vi "ex_createorOpenTDM.vi"(0 "file path in":path, 1 "overwrite_mode_multi":T3(ring), 2 "overwrite_mode":T4(ring), 3 "append info in":T5, 4 "file dialog?":bool, 5 "error in (no error)":errorcluster, 6 "file params":T1 {"Flags"."time preference" items=["Absolute", "Relative"]; "Flags"."x_columns" items=["None", "One", "Multiple"]; "origin time" format="%<%X\n%x>T"}, 7 "multi_file":bool, 9 "new file?":bool, 11 "Simulate Non-First Call":bool) -> (13 "new file was created":bool, 14 "file path out":path, 15 "dialog was cancelled":bool, 16 "keep loop going":bool, 17 "append info out":T5, 18 "file params out":T1 {"Flags"."time preference" items=["Absolute", "Relative"]; "Flags"."x_columns" items=["None", "One", "Multiple"]; "origin time" format="%<%X\n%x>T"}, 19 "error out":errorcluster)   [LabVIEW 2017]
uses:
  <vilib>/Platform/express/TDMExpress.llb/ex_appendInfoTDM.ctl
  <vilib>/express/express output/ExFileWriteBlock.llb/ex_WriteFileParams.ctl
  <vilib>/express/express input/ExFileReadBlock.llb/ex_ReadFileParams.ctl
  <vilib>/Platform/storage/lvStorage.llb/_openFunction.ctl
  <vilib>/express/express shared/ExFile.llb/ex_FileFormatSelector.ctl
  <vilib>/express/express shared/ExFile.llb/ex_FileGlobals.vi
  <vilib>/Platform/storage/Storage.llb/__closeStorageFromObject.vi
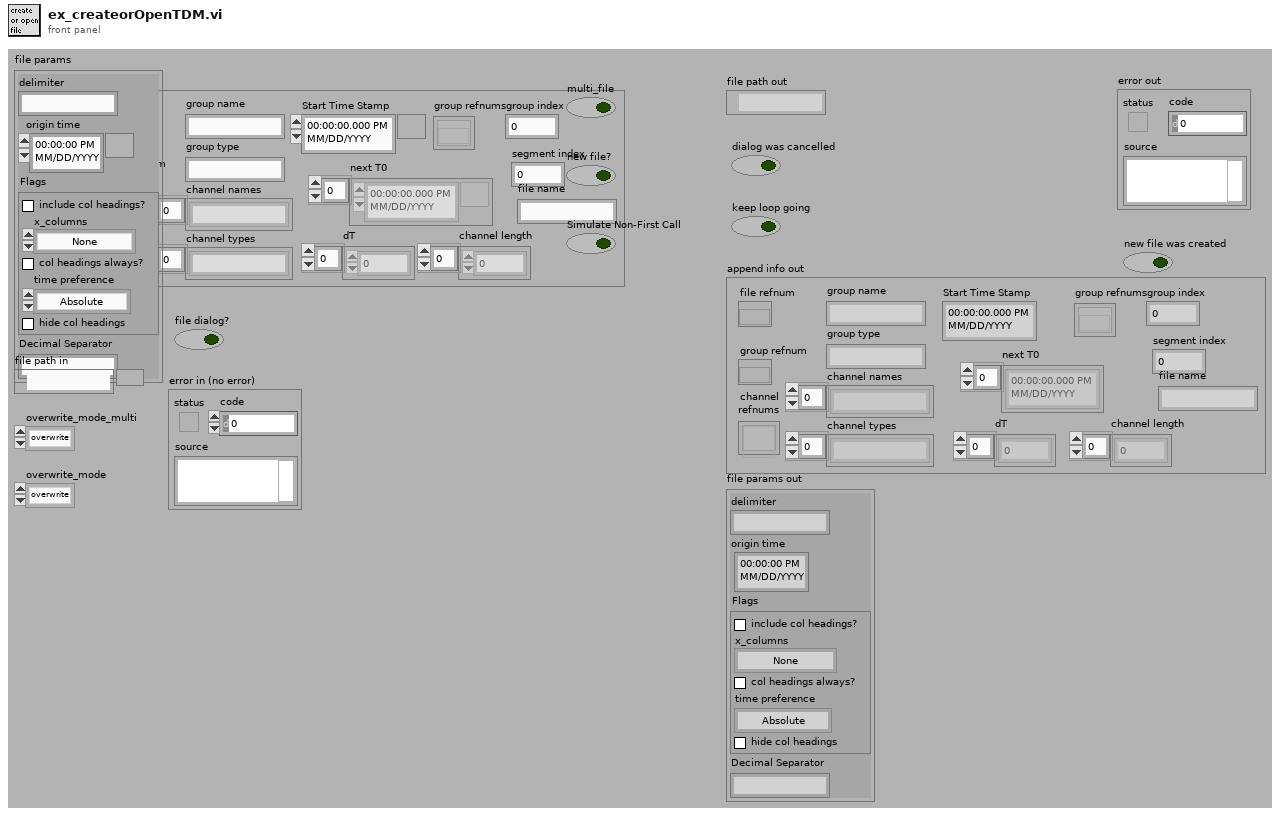
[diagram p1: front panel]
types:
  T1 = typedef "ex_WriteFileParams.ctl" = cluster{"delimiter":string, "origin time":timestamp, "Flags":T2, "Decimal Separator":string}
  T2 = typedef "ex_ReadFileParams.ctl" = cluster{"include col headings?":bool, "x_columns":u16, "col headings always?":bool, "time preference":u16, "hide col headings":bool}
  T3 = enum16{"overwrite", "overwrite & backup", "next avail"}
  T4 = enum16{"overwrite", "overwrite & backup", "append", "next avail"}
  T5 = typedef "ex_appendInfoTDM.ctl" = cluster{"channel\nrefnums":refnum<k20>[], "channel names":string[], "channel types":string[], "file refnum":refnum<k20>, "group refnum":refnum<k20>, "group name":string, "group type":string, "next T0":timestamp[], "dT":dbl[], "Start Time Stamp":timestamp, "channel length":u32[], "group index":u32, "group refnums":refnum<k20>[], "file name":string, "segment index":u32}
  T6 = typedef "ex_FileFormatSelector.ctl" = enum32{"lvm", "tdm", "other"}
  T7 = typedef "_openFunction.ctl" = enum16{"open", "open or create", "create or replace", "create", "open (read only)"}
  T8 = enum16{"existing file", "new file", "new or existing file", "existing dir", "new dir", "new or existing dir", "existing file (use LLBs)", "new file (use LLBs)", "new or existing file (use LLBs)", "new or existing file or directory (use LLBs)"}
  T9 = cluster{"message":string, "T button name":string, "F button name":string}
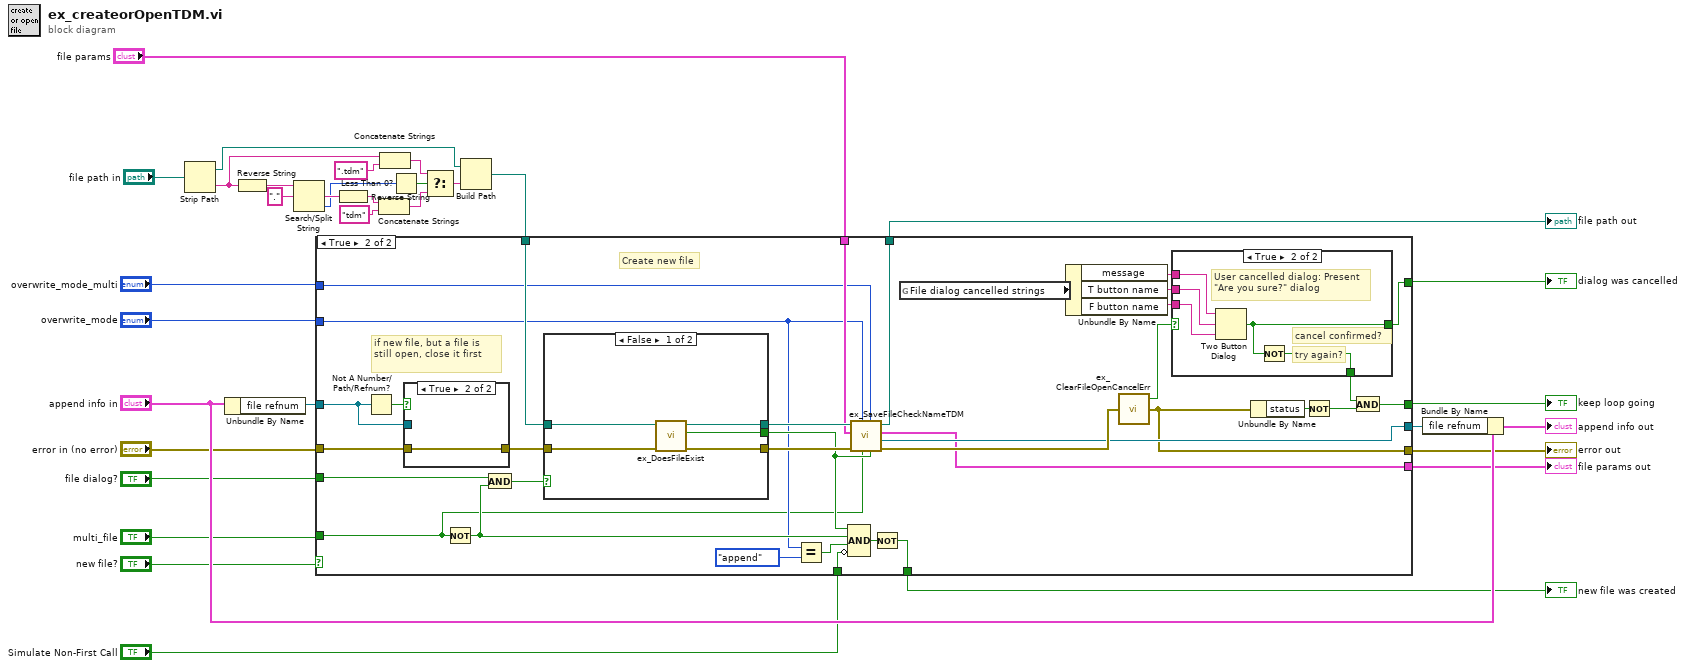
[diagram p0: block diagram]
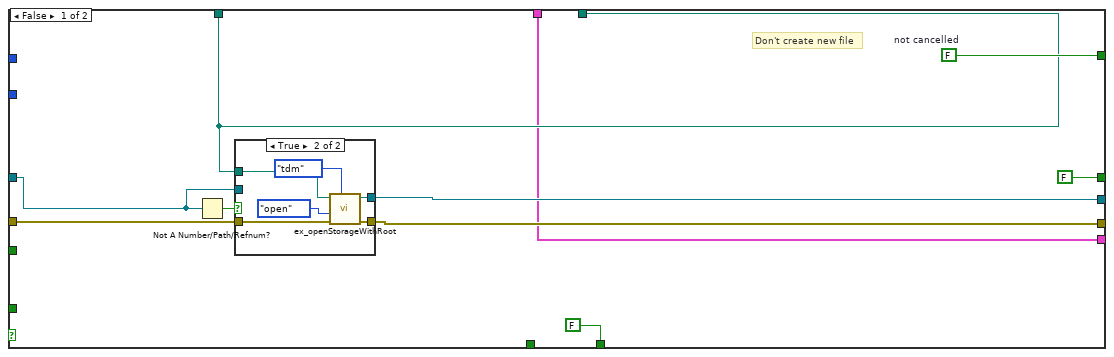
[diagram p2: hidden frame]
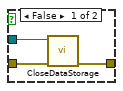
[diagram p4: hidden frame]
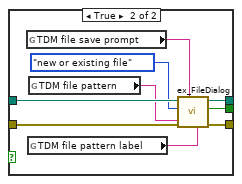
[diagram p6: hidden frame]
diagram:
  n1 = Strip Path(path="file path in") -> (stripped path=w3:path, name=w5:string)
  n2 = Unbundle By Name("append info in") -> ("file refnum"=w28:refnum<k20>)
  n3 = Reverse String(1:w5) -> (0:w15:string)
  n4 = Search/Split String(string=w15, search string/char (-)=".") -> (match + rest of string=w13:string, offset of match=w10:i32)  [unwired: 2 out]
  n5 = Reverse String(1:w13) -> (0:w11:string)
  n6 = Concatenate Strings(w11, "tdm" ("replace string (\"\")")) -> (w6:string)
  n7 = Concatenate Strings(w5, ".tdm" ("replace string (\"\")")) -> (w7:string)
  n8 = Less Than 0?(x=w10) -> (x < 0?=w9:bool)
  n9 = Select(t=w7, s=w9, f=w6) -> (s? t:f=w4:string)
  n10 = Build Path(base path=w3, name or relative path=w4) -> (appended path=w1:path)
  n11 = case shown="True" "new file?" {
    tunnel: "error in (no error)" -> [w40 w58]
    tunnel: w1 -> [w37 w78]
    tunnel: [w39 w61] -> w26
    tunnel: [w34 w53] -> w27
    tunnel: "Simulate Non-First Call" -> [_ w76]
    tunnel: [w43 w72] -> w24
    tunnel: [FALSE w71] -> w30
    tunnel: [w38 w68] -> w32
    tunnel: "file params" -> [w34 w67]
    tunnel: "multi_file" -> [_ w52]
    tunnel: "file dialog?" -> [_ w66]
    tunnel: "overwrite_mode_multi" -> [_ w65]
    tunnel: "overwrite_mode" -> [_ w64]
    tunnel: [FALSE w59] -> w23
    tunnel: w28 -> [w35 w55]
    tunnel: [w37 w54] -> w25
    frame False {
      w43 = FALSE  # not cancelled
      # "Don't create new file"
      n12 = Not A Number/Path/Refnum?(number/path/refnum=w35) -> (NaN/Path/Refnum?=w36:bool)
      n13 = case shown="True" w36 {
        tunnel: w40 -> [w45 w50]
        tunnel: [w45 w49] -> w39
        tunnel: [w44 w48] -> w38
        tunnel: w37 -> [_ w47]
        tunnel: w35 -> [w44 _]
        frame False {
        }
        frame True {
          n14 = call <vilib>:"ex_openStorageWithRoot.vi"("storage_format"=ex_FileFormatSelector."tdm", "error in (no error)"=w50, "Overwrite Options"=_openFunction."open", "Storage Location"=w47) -> ("error out"=w49:errorcluster, "Data Object"=w48:refnum<k20>)  [unwired: 1 in, 5 out]
        }
      }
    }
    frame True {
      # "if new file, but a file is still open, close it first"
      # "Create new file"
      n15 = Not A Number/Path/Refnum?(number/path/refnum=w55) -> (NaN/Path/Refnum?=w56:bool)
      n16 = case shown="True" w56 {
        tunnel: w58 -> [w89 w90]
        tunnel: [w88 w90] -> w57
        tunnel: w55 -> [w87 _]
        frame False {
          n17 = call-poly <vilib>:"CloseDataStorage.vi"("error in (no error)"=w89, "storage refnum"=w87) -> ("error out"=w88:errorcluster)  [unwired: 5 out]
        }
        frame True {
        }
      }
      n18 = Not(x=w52) -> (.not. x?=w86:bool)
      n19 = And(x=w66, y=w86) -> (x .and. y?=w85:bool)
      n20 = case shown="False" w85 {
        tunnel: w78 -> [w100 w110]
        tunnel: [w99 w109] -> w74
        tunnel: [w98 w108] -> w75
        tunnel: w57 -> [w101 w107]
        tunnel: [w97 w106] -> w73
        frame False {
          n21 = call <vilib>:"ex_DoesFileExist.vi"("error in"=w101, "file path"=w100) -> ("error out"=w98:errorcluster, "file exists"=w97:bool, "dup file path"=w99:path)  [unwired: 3 out]
        }
        frame True {
          n22 = global read "ex_FileGlobals.vi" "TDM file save prompt"() -> (w104:string)
          n23 = global read "ex_FileGlobals.vi" "TDM file pattern label"() -> (w103:string)
          n24 = global read "ex_FileGlobals.vi" "TDM file pattern"() -> (w102:string)
          n25 = call <vilib>:"ex_FileDialog.vi"("pattern label"=w103, "pattern"=w102, "prompt"=w104, "error in (no error)"=w107, "select mode"=T8."new or existing file", "start path"=w110) -> ("error out"=w108:errorcluster, "file exists?"=w106:bool, "selected file path"=w109:path)  [unwired: 3 out]
        }
      }
      n26 = Equal?(x=w64, y=T4."append" ("overwrite_mode")) -> (x = y?=w80:bool)
      n27 = Compound Arithmetic op=AND(w73, w86, w80, invert w76) -> (w79:bool)
      n28 = call <vilib>:"ex_SaveFileCheckNameTDM.vi"("file exists?"=w73, "overwrite_mode_multi"=w65, "multi_file"=w52, "overwrite_mode"=w64, "error in (no error)"=w75, "file params in"=w67, "file path"=w74) -> ("error out"=w70:errorcluster, "Storage RefNum"=w68:refnum<k20>, "file params out"=w53:T1, "file path out"=w54:path)  [unwired: 1 out]
      n29 = Not(x=w79) -> (.not. x?=w71:bool)
      n30 = global read "ex_FileGlobals.vi" "File dialog cancelled strings"() -> (w77:T9)
      n31 = Unbundle By Name(w77) -> ("message"=w84:string, "T button name"=w83:string, "F button name"=w82:string)
      n32 = call <vilib>:"ex_ClearFileOpenCancelErr.vi"("error in"=w70) -> ("error out"=w61:errorcluster, "cancelled?"=w69:bool)  [unwired: 3 out]
      n33 = case shown="True" w69 {
        selector: w69 -> [w91 _]
        tunnel: w82 -> [_ w96]
        tunnel: w84 -> [_ w95]
        tunnel: w83 -> [_ w94]
        tunnel: [w91 w93] -> w72
        tunnel: [w91 w92] -> w60
        frame False {
          # "not cancelled"
          # "file dialog not cancelled"
        }
        frame True {
          # "cancel confirmed?"
          # "try again?"
          # "User cancelled dialog: Present\n\"Are you sure?\" dialog"
          n34 = Two Button Dialog(message=w95, 1:w96, 2:w94) -> (T button?=w93:bool)
          n35 = Not(x=w93) -> (.not. x?=w92:bool)
        }
      }
      n36 = Unbundle By Name(w61) -> ("status"=w62:bool)
      n37 = Not(x=w62) -> (.not. x?=w63:bool)
      n38 = And(x=w60, y=w63) -> (x .and. y?=w59:bool)
    }
  }
  "new file was created" <- w30
  "file params out" <- w27
  "error out" <- w26
  "file path out" <- w25
  "dialog was cancelled" <- w24
  "keep loop going" <- w23
  n39 = Bundle By Name(cluster="append info in", "file refnum"=w32) -> (→"append info out":T5)
